vi "GetFirstAndAllRowsOfOfficialRes.vi"(11 "file (use dialog)":path=path "/Users/blagojnikolov/Desktop/@tmp/fromSite.txt") -> (0 "All Officials Result":dbl[][](array[numeric]), 1 "text":string, 3 "First Row":dbl[](array[numeric]))   [LabVIEW 2023]
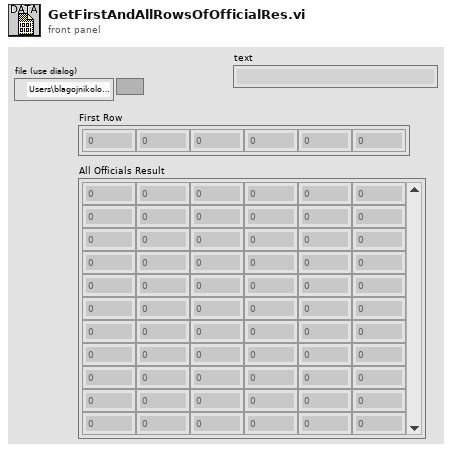
[diagram p1: front panel]
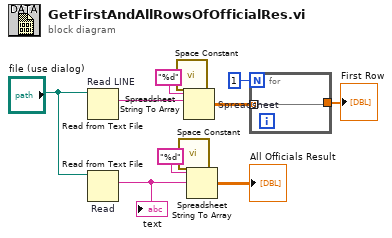
[diagram p0: block diagram]
diagram:
  n1 = Read from Text File "Read LINE"(file (use dialog)="file (use dialog)") -> (text=w11:string)  [unwired: 3 in, 3 out]
  n2 = Read from Text File "Read"(file (use dialog)="file (use dialog)") -> (text=w1:string)  [unwired: 3 in, 3 out]
  "text" <- w1
  n3 = call <vilib>:"Space Constant.vi"() -> ("String"=w9:string)
  n4 = call <vilib>:"Space Constant.vi"() -> ("String"=w5:string)
  n5 = Spreadsheet String To Array "Spreadsheet"(delimiter (Tab)=w9, format string="%d", spreadsheet string=w11) -> (array=w8:dbl[][])  [unwired: 1 in]
  n6 = Spreadsheet String To Array(delimiter (Tab)=w5, format string="%d", spreadsheet string=w1) -> (array=→"All Officials Result":dbl[][])  [unwired: 1 in]
  n7 = for {
    N: 1 -> [_]
    tunnel: w8 -> [w12] mode=indexing
    tunnel: [w12] -> w6
  }
  "First Row" <- w6
